vi "Set FC1.vi"(10 "FC1":refnum<class "Actuator Cylinder.lvclass">, 11 "SingleCylinderActuator in":refnum<class "Single Cylinder Actuator.lvclass">) -> (3 "SingleCylinderActuator out":refnum<class "Single Cylinder Actuator.lvclass">)   [LabVIEW 2015, in "Single Cylinder Actuator.lvclass"]
uses:
  Single Cylinder Actuator.lvclass
  Actuator Cylinder/Actuator Cylinder/Actuator Cylinder.lvclass
  Single Cylinder Actuator.lvclass/Single Cylinder Actuator.ctl
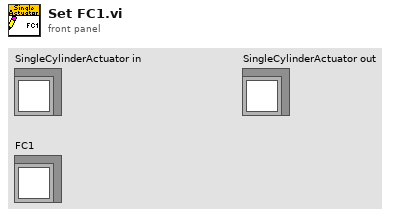
[diagram p1: front panel]
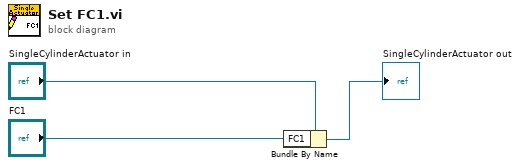
[diagram p0: block diagram]
diagram:
  n1 = Bundle By Name(cluster="SingleCylinderActuator in", "FC1"="FC1") -> (→"SingleCylinderActuator out":refnum<class "Single Cylinder Actuator.lvclass">)
